vi "Simple AAV using Express VI.vi"() -> ()   [LabVIEW 2022 SP3]
panel:
  out "Waveform Graph":dynamicdata(graph)
  out "Numeric Indicator":dbl
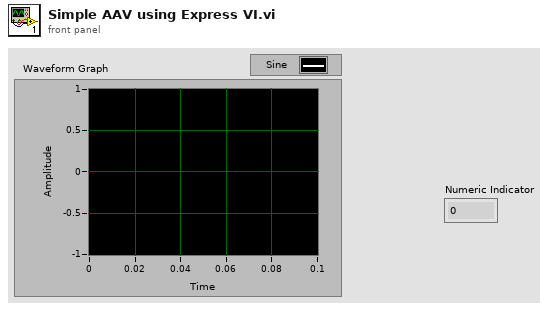
[diagram p1: front panel]
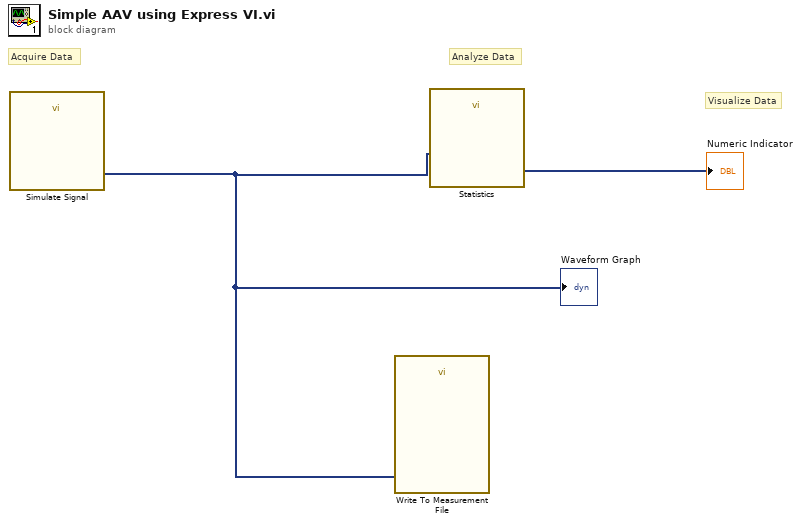
[diagram p0: block diagram]
diagram:
  # "Visualize Data"
  # "Analyze Data"
  # "Acquire Data"
  n1 = call "Simulate Signal"() -> ("Sine"=w1:dynamicdata)  [unwired: 14 in, 1 out]
  "Waveform Graph" <- w1
  n2 = call "Write To Measurement File"("Signals"=w1) -> ()  [unwired: 16 in, 3 out]
  n3 = call "Statistics"("Signals"=w1) -> ("Arithmetic Mean"=→"Numeric Indicator":dynamicdata)  [unwired: 25 in, 1 out]
